vi "SIM evaluate interpolating polynomial.vi"(6 "interp poly order":i32, 8 "time to evalulate":dbl, 9 "current time":dbl, 10 "timestep":dbl, 11 "Backward differences":dbl[][](array[numeric])) -> (3 "result":dbl[](array[numeric]))   [LabVIEW 2018]
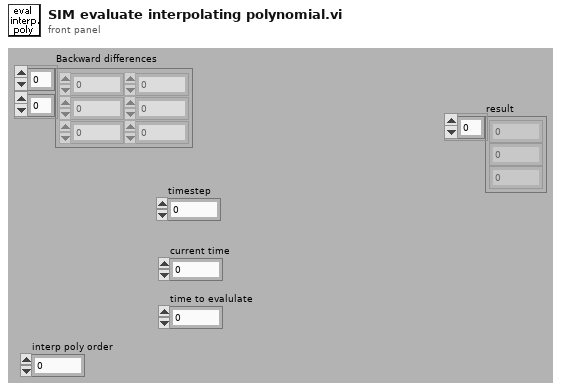
[diagram p1: front panel]
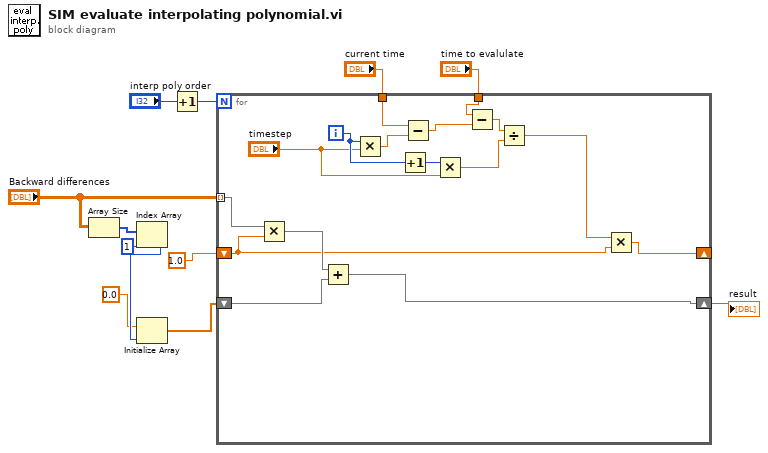
[diagram p0: block diagram]
diagram:
  n1 = Array Size(array="Backward differences") -> (size(s)=w10:i32[])
  n2 = Index Array(array=w10, index=1) -> (element=w9:i32)
  n3 = Initialize Array(0.0, w9) -> (w7:dbl[])
  n4 = Increment(x="interp poly order") -> (x+1=w1:i32)
  n5 = for {
    N: w1 -> [_]
    tunnel: "Backward differences" -> [w28] mode=indexing
    shift-right: [w13] -> _
    shift-left: 1.0 -> [w15]
    shift-right: [w25] -> w3
    shift-left: w7 -> [w26]
    tunnel: "current time" -> [w23]
    tunnel: "time to evalulate" -> [w22]
    i -> [w19]
    n6 = Multiply(x=w28, y=w15) -> (x*y=w27:dbl[])
    n7 = Add(x=w27, y=w26) -> (x+y=w25:dbl[])
    n8 = Multiply(x=w19, y="timestep") -> (x*y=w24:dbl)
    n9 = Increment(x=w19) -> (x+1=w17:i32)
    n10 = Subtract(x=w23, y=w24) -> (x-y=w21:dbl)
    n11 = Multiply(x=w17, y="timestep") -> (x*y=w16:dbl)
    n12 = Subtract(x=w22, y=w21) -> (x-y=w20:dbl)
    n13 = Divide(x=w20, y=w16) -> (x/y=w14:dbl)
    n14 = Multiply(x=w14, y=w15) -> (x*y=w13:dbl)
  }
  "result" <- w3
